vi "Drive Away from Obstacle.vi"(5 "max reverse velocity (m/s)":dbl, 7 "max angular velocity (rad/s)":dbl=1.0, 8 "error in (no error)":errorcluster, 11 "gap":T1) -> (0 "error out":errorcluster, 2 "steering frame velocity":dbl[](array[numeric]))   [LabVIEW 2014]
doc: "Sets the steering frame velocity so that the robot moves in reverse and rotates towards the gap."
uses:
  <vilib>/robotics/Obstacle Avoidance/Simple Vector Field Histogram/Gap Description.ctl
  <vilib>/robotics/Obstacle Avoidance/Simple Vector Field Histogram/NI_Robotics_Simple Vector Field Histogram.lvlib
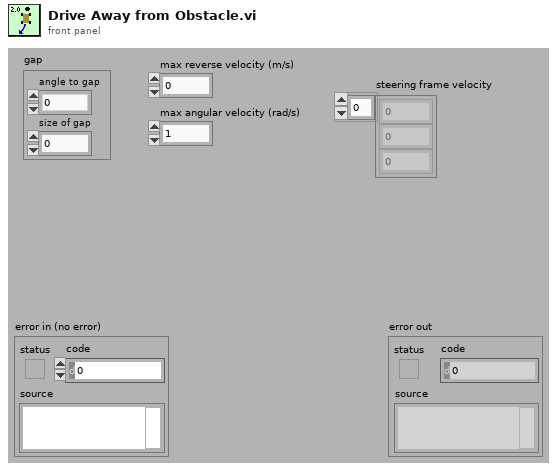
[diagram p1: front panel]
types:
  T1 = typedef "NI_Robotics_Simple Vector Field Histogram.lvlib/Gap Description.ctl" = cluster{"angle to gap":dbl, "size of gap":dbl}
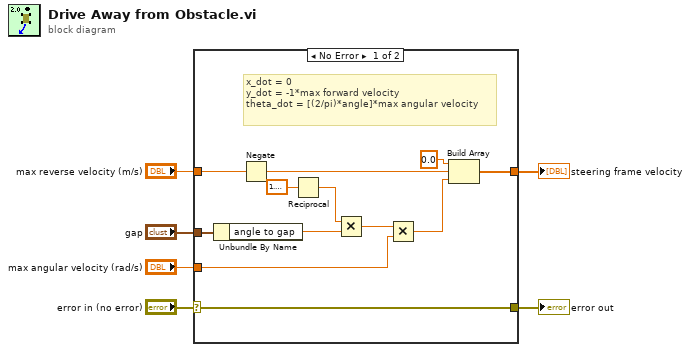
[diagram p0: block diagram]
diagram:
  n1 = case shown="No Error" "error in (no error)" {
    selector: "error in (no error)" -> [w18 w19]
    tunnel: "gap" -> [w17 _]
    tunnel: [w18 w19] -> w4
    tunnel: "max reverse velocity (m/s)" -> [w14 _]
    tunnel: "max angular velocity (rad/s)" -> [w8 _]
    tunnel: [w15 _] -> w1
    frame No Error {
      # "x_dot = 0\ny_dot = -1*max forward velocity\ntheta_dot = [(2/pi)*angle]*max angular velocity"
      n2 = Unbundle By Name(w17) -> ("angle to gap"=w11:dbl)
      n3 = Negate(x=w14) -> (-x=w13:dbl)
      n4 = Reciprocal(x=1.5707963267948966) -> (1/x=w10:dbl)
      n5 = Multiply(x=w10, y=w11) -> (x*y=w9:dbl)
      n6 = Multiply(x=w9, y=w8) -> (x*y=w7:dbl)
      n7 = Build Array(0.0 ("element"), w13, w7) -> (w15:dbl[])
    }
    frame Error {
    }
  }
  "error out" <- w4
  "steering frame velocity" <- w1
